vi "Channel GUIDs.vi"() -> ()   [LabVIEW 2017, in "Modules.lvlib" / "RSI Module.lvclass"]
uses:
  RSI Module.lvclass
panel:
  in  "Module Config Channel":string="9888E34F-1DAF-F5F9-23C9-A92C2C9D9594"
  in  "Module Config Section":string="1598AB10-D25A-B2C1-00CA-EA7BE52FA7ED"
  in  "AI Channel":string="7D1F352D-C320-52BF-1ACF-10488F36F94D"
  in  "AO Channel":string="A613CB09-4F09-9982-AF75-BF47F7A4882F"
  in  "DI Channel":string="F233E90F-ECCA-EF6E-8EEB-159F82DA778F"
  in  "DO Channel":string="F43DA51B-9C6C-5797-56DC-ED47295D1D2E"
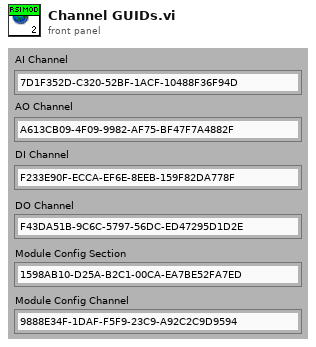
[diagram p1: front panel]
diagram:
